vi "Send Message To Host [OUT].vi"(7 "Micropulse # In":i32, 8 "error in (no error)":errorcluster, 9 "Parameter":u8 caption="Parameter (0-255)", 10 "Header No.":u8=6 caption="Header No. (def: 0x6)" format="%02x") -> (0 "error out":errorcluster, 5 "Micropulse # Out":i32)   [LabVIEW 2026, in "MicroPulse_Driver.lvlib"]
doc: "To program action on axis condition.\n\nFormat : MSE <axis> <mode> [off]\n\nDescription :\nThis command works in the same way as INE in that the command line following the MSE command is stored and invoked when the specified condition occurs. There are four such conditions corresponding to different events at the end of the axis move or inspection commands (MOV, MRE or FLY). In particular the programmed command line may redefine the MSE setting. If MSE is disabled, then MicroPulse defaults to its normal mode of sending LLC message to host on any axis stop.\n\nNOTE :\nIt MUST be set before any other motor commands are used. It is usual to set this command once only at power-up.\n\nParameters:\n<axis> : Axis number 1 to 4\n\n<mode> :\n0 normal stop\n1 end of FLR or FLZ\n2 stall\n3 overshoot\n4 any axis stop\n\n[off] : Optional. If this parameter is omitted the function is enabled.\n\nExample : Causes CER 10 message when axis 2 stalls\nMSE 2 2\nOUT 6 10\n\nSystem Compatibility:\nModes 0, 3 and 4 are only available with MicroPulse 5 with motor controller option fitted."
uses:
  MicroPulse_Driver.lvlib
  Private/MP-Registry Action-Enum.ctl
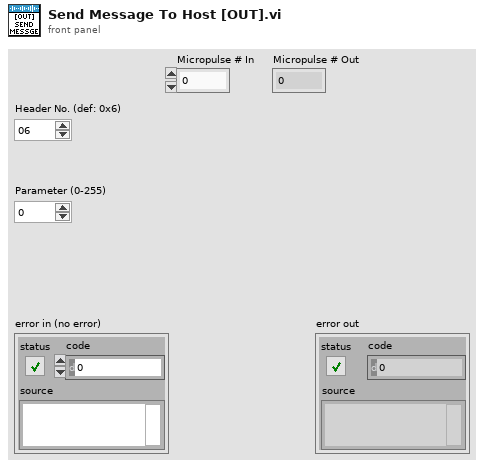
[diagram p1: front panel]
types:
  T1 = typedef "MicroPulse_Driver.lvlib/MP-Registry Action-Enum.ctl" = enum16{"Read", "Add Test", "Add Command", "Add Gate Command", "Add Encoder Command", "Clear Command  List", "Set Registry", "Set System Details", "Set DOF", "Set Velocity", "Disable Asynch Reads", "Enable Asynch Reads", "Add Connection", "Disconnect", "Shutdown"}
  T2 = typedef "Micropulse.lvlib/TCP config.ctl" = cluster{"Connection ID":refnum<k5>, "IP address":string, "host port":u16, "OC timeout":i32, "Read timeout":i32, "Write timeout":i32}
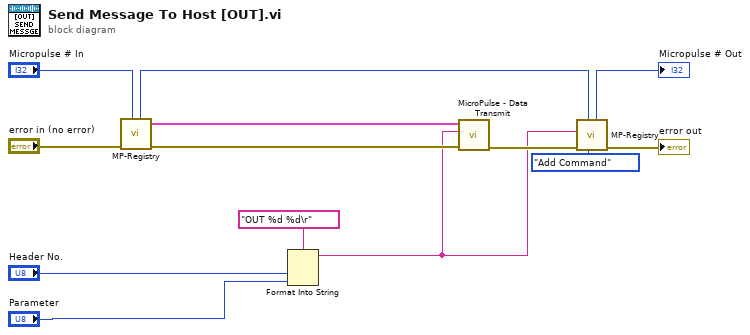
[diagram p0: block diagram]
diagram:
  n1 = call "MP-Registry.vi"("Micropulse # In"="Micropulse # In", "error in (no error)"="error in (no error)") -> ("error out"=w11:errorcluster, "TCP config"=w10:T2, "Micropulse # Out"=w7:i32)  [unwired: 6 in, 1 out]
  n2 = Format Into String(format string="OUT %d %d\r", "Header No.", "Parameter") -> (resulting string=w4:string)  [unwired: 2 in, 1 out]
  n3 = call "MicroPulse - Data Transmit.vi"("error in (no error)"=w11, "data"=w4, "TCP config"=w10) -> ("error out"=w8:errorcluster)  [unwired: 6 in, 2 out]
  n4 = call "MP-Registry.vi"("Action"=MP-Registry_Action-Enum."Add Command", "Micropulse # In"=w7, "error in (no error)"=w8, "Data in"=w4) -> ("error out"=→"error out":errorcluster, "Micropulse # Out"=→"Micropulse # Out":i32)  [unwired: 4 in, 2 out]
